vi "Set_Parameter_Instrument (Json).vi"(8 "error in (no error)":errorcluster caption="entrée d'erreur (pas d'erreur)", 10 "Parameter (Json)":string, 11 "Flash_SIN_FP en entrée":refnum<class "Flash_SIN_FP.lvclass">) -> (0 "error out":errorcluster caption="sortie d'erreur", 3 "Flash_SIN_FP en sortie":refnum<class "Flash_SIN_FP.lvclass">)   [LabVIEW 2020, in "Library Test.lvlib" / "Flash_SIN_FP.lvclass"]
uses:
  Flash_SIN_FP.lvclass
  C:/Users/ngarcin/OneDrive - Altyor/Standard TB/Suite TB45/Class/Test/Test (Default)/Test (Default).lvclass
  C:/Users/ngarcin/OneDrive - Altyor/Standard TB/Suite TB45/Class/Test/Flash_Commander/Flash_Commander.lvclass
  Commun VI/TypeDef/Variable Printable.ctl
  Flash_SIN_FP.lvclass/Flash_SIN_FP.ctl
  JSON API/JSON Value/Set from JSON string.vi
  Flash_Commander/Flash_Commander.lvclass
  JSON API/JSON Value/JSON Value.lvclass
  JSON API/Variant JSON/Variant JSON.lvlib
  JSON API/Get Polymorphic/JSON GetSet.lvlib
  Commun VI/Library Commun.lvlib
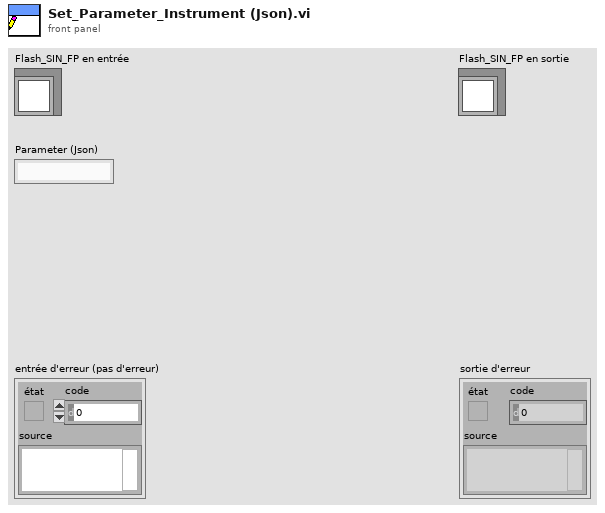
[diagram p1: front panel]
types:
  T1 = enum16{"Get Variable", "Get All Variables", "Set Variable", "Delete Variable", "Delete All Variable"}
  T2 = typedef "Variable Printable.ctl" = string
  T3 = cluster{"Bootloader path":path, "Firmware path":path, "Security path":path, "commander path":path, "Bat path":path}
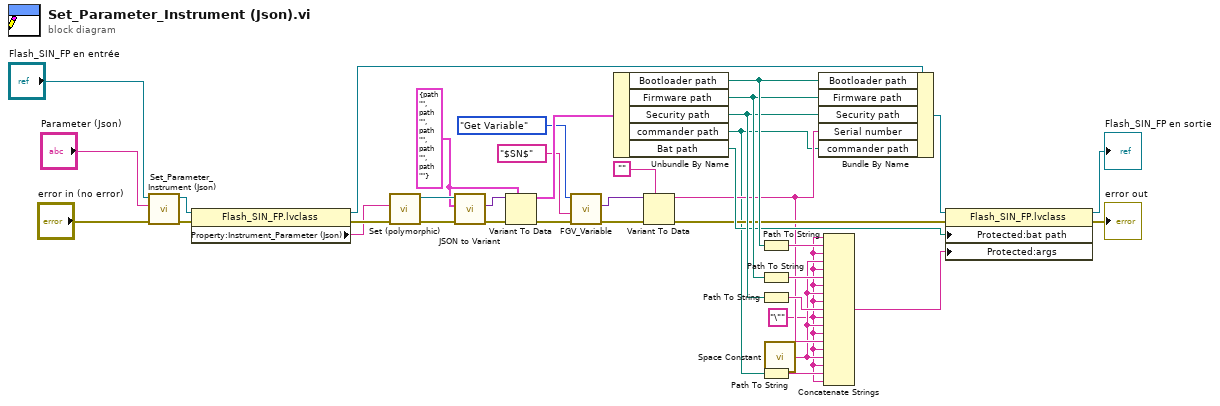
[diagram p0: block diagram]
diagram:
  w1 = "\""
  w24 = T3 {"Bootloader path"=path "", "Firmware path"=path "", "Security path"=path "", "commander path"=path "", "Bat path"=path ""} ("Cluster des données privées de classe")
  n1 = call-parent "Set_Parameter_Instrument (Json).vi"("error in (no error)"="error in (no error)", "Parameter (Json)"="Parameter (Json)", "Test (Default) en entrée"="Flash_SIN_FP en entrée") -> ("error out"=w32:errorcluster, "Test (Default) en sortie"=w31:refnum<class "Flash_SIN_FP.lvclass">)  [unwired: 7 in]
  n2 = property class="Flash_SIN_FP.lvclass"(reference=w31, error in=w32) -> (reference out=w27:refnum<class "Flash_SIN_FP.lvclass">, error out=w30:errorcluster, "Property:Instrument_Parameter (Json)"=w28:string)
  n3 = call-poly "Set (polymorphic).vi"("error in (no error)"=w30, "JSON stream"=w28) -> ("error out"=w35:errorcluster, "JSON Value out"=w37:refnum<class "JSON Value.lvclass">)  [unwired: 7 in, 1 out]
  n4 = call "JSON to Variant.vi"("error in (no error)"=w35, "Variant (Data Type)"=w24, "JSON Value"=w37) -> ("error out"=w36:errorcluster, "Variant out"=w34:variant)  [unwired: 7 in]
  n5 = Variant To Data(error in=w36, type=w24, Variant=w34) -> (data=w26:T3, error out=w9:errorcluster)
  n6 = call "FGV_Variable.vi"("error in (no error)"=w9, "Variable"=T2 "$SN$" ("Variable Printable"), "Function"=T1."Get Variable") -> ("error out"=w10:errorcluster, "Data Out"=w6:variant)  [unwired: 6 in, 1 out]
  n7 = Unbundle By Name(w26) -> ("Bootloader path"=w17:path, "Firmware path"=w16:path, "Security path"=w15:path, "commander path"=w2:path, "Bat path"=w14:path)
  n8 = Variant To Data(error in=w10, type="", Variant=w6) -> (data=w5:string, error out=w8:errorcluster)
  n9 = Path To String(path=w17) -> (string=w20:string)
  n10 = Path To String(path=w16) -> (string=w19:string)
  n11 = Path To String(path=w15) -> (string=w18:string)
  n12 = Path To String(path=w2) -> (string=w3:string)
  n13 = call <vilib>:"Space Constant.vi"() -> ("String"=w4:string)
  n14 = Bundle By Name(cluster=w27, "Bootloader path"=w17, "Firmware path"=w16, "Security path"=w15, "Serial number"=w5, "commander path"=w2) -> (w23:refnum<class "Flash_SIN_FP.lvclass">)
  n15 = Concatenate Strings(w1, w20, w1, w4, w1, w19, w1, w4, w1, w18, w1, w4, w1, w5, w1, w4, w1, w3, w1) -> (w13:string)
  n16 = property class="Flash_SIN_FP.lvclass"(reference=w23, error in=w8, "Protected:bat path"=w14, "Protected:args"=w13) -> (reference out=→"Flash_SIN_FP en sortie":refnum<class "Flash_SIN_FP.lvclass">, error out=→"error out":errorcluster)
